vi "Bottom Empty Slot.vi"(11 "Room":string[](array[string])) -> (3 "Slot":i32)   [LabVIEW 2019, in "23.lvlib"]
uses:
  23.lvlib
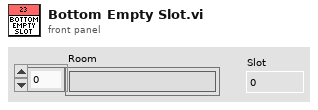
[diagram p1: front panel]
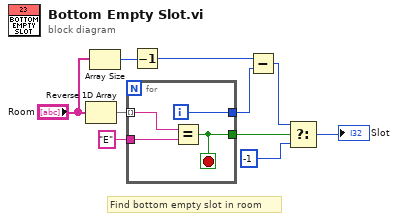
[diagram p0: block diagram]
diagram:
  # "Find bottom empty slot in room"
  n1 = Reverse 1D Array(array="Room") -> (reversed array=w6:string[])
  n2 = Array Size(array="Room") -> (size(s)=w4:i32)
  n3 = for {
    tunnel: w6 -> [w14] mode=indexing
    tunnel: "E" ("y") -> [w13]
    tunnel: [w12] -> w2
    tunnel: [w11] -> w8
    i -> [w12]
    stop <- w11 stop-if-true
    n4 = Equal?(x=w14, y=w13) -> (x = y?=w11:bool)
  }
  n5 = Decrement(x=w4) -> (x-1=w3:i32)
  n6 = Subtract(x=w3, y=w2) -> (x-y=w1:i32)
  n7 = Select(t=w1, s=w8, f=-1) -> (s? t:f=→"Slot":i32)
